vi "Check the Symbols.vi"(0 "Item Symbols":i32[](array[numeric])) -> (4 "All Selected?":bool, 6 "None Selected":bool)   [LabVIEW 2021, in "Measurement Builder.lvlib"]
uses:
  Measurement Builder.lvlib
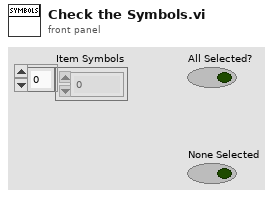
[diagram p1: front panel]
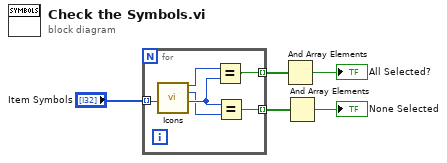
[diagram p0: block diagram]
diagram:
  n1 = for {
    tunnel: "Item Symbols" -> [w10] mode=indexing
    tunnel: [w9] -> w2 mode=indexing
    tunnel: [w8] -> w3 mode=indexing
    n2 = call "Icons.vi"() -> ("Selected"=w7:i32, "Non Selected"=w6:i32)  [unwired: 14 in]
    n3 = Equal?(x=w7, y=w10) -> (x = y?=w9:bool)
    n4 = Equal?(x=w10, y=w6) -> (x = y?=w8:bool)
  }
  n5 = And Array Elements(Boolean array=w2) -> (logical AND=→"All Selected?":bool)
  n6 = And Array Elements(Boolean array=w3) -> (logical AND=→"None Selected":bool)
